vi "Ping.vi"(1 "IP Address":string) -> (0 "Found?":bool)   [LabVIEW 2018]
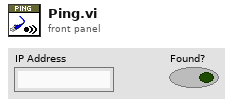
[diagram p1: front panel]
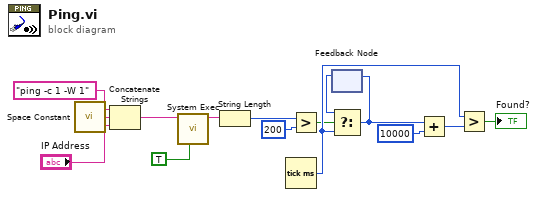
[diagram p0: block diagram]
diagram:
  n1 = call <vilib>:"Space Constant.vi"() -> ("String"=w4:string)
  n2 = Concatenate Strings("ping -c 1 -W 1" ("command line"), w4, "IP Address") -> (w2:string)
  n3 = call <vilib>:"System Exec.vi"("run minimized? (F)"=TRUE, "command line"=w2) -> ("standard output"=w5:string)  [unwired: 6 in, 3 out]
  n4 = String Length(string=w5) -> (length=w6:i32)
  n5 = Tick Count (ms)() -> (millisecond timer value=w15:u32)
  n6 = Greater?(x=w6, y=200) -> (0:w9:bool)
  n7 = feedback #1() -> (w10:u32)  [unwired: 1 in]
  n8 = Select(t=w10, s=w9, f=w15) -> (s? t:f=w11:u32)
  n9 = feedback-in #1(w11) -> ()
  n10 = Add(x=w11, y=u32 10000) -> (x+y=w12:u32)
  n11 = Greater?(x=w15, y=w12) -> (0:→"Found?":bool)
